vi "反控参数设置.vi"(8 "value time":timestamp, 9 "value float":sgl, 10 "设置参数":T2(ring)=enum."CODMn", 11 "设置类型":T1(ring)=enum."i13002") -> ()   [LabVIEW 2016]
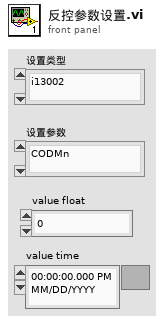
[diagram p1: front panel]
types:
  T1 = enum16{"i13001", "i13002", "i13003", "i13004", "i13005", "i13006", "i13007", "i13008", "i13009", "i13010", "i13011", "i13012", "i13013", "i13014", "i13015", "i13016", "i13017", "i13101", "i13102", "i13103", "i13104", "i13105", "i13106", "i13107", "i13108", "i13109", "i13110"}
  T2 = enum16{"", "CODMn", "PH", "氨氮", "总氮", "总磷", "CODCr", "电导率", "水温", "溶解氧", "浊度", "叶绿素", "藻密度", "ORP"}
  T3 = cluster{"status":bool, "代码":u16, "source":string}
  T4 = cluster{"测量量程":dbl, "测量精度":dbl, "测量间隔":dbl, "消解温度":dbl, "消解时长":dbl, "空白校准时间":timestamp, "曲线截距":dbl, "曲线斜率":dbl, "测量检出限":dbl, "测量信号值":dbl, "线性相关系数":dbl, "二次多项式系数":dbl, "标样校准时间":timestamp, "稀释倍数":dbl, "三项式系数":dbl, "空白标定系数":dbl, "量程系数":dbl, "F0/ORPA":dbl, "F1/ORPB":dbl, "F2/ORPK":dbl, "F3":dbl, "F4":dbl, "F5":dbl, "F6":dbl, "F7":dbl, "X0/滴定数":dbl, "量程":dbl}
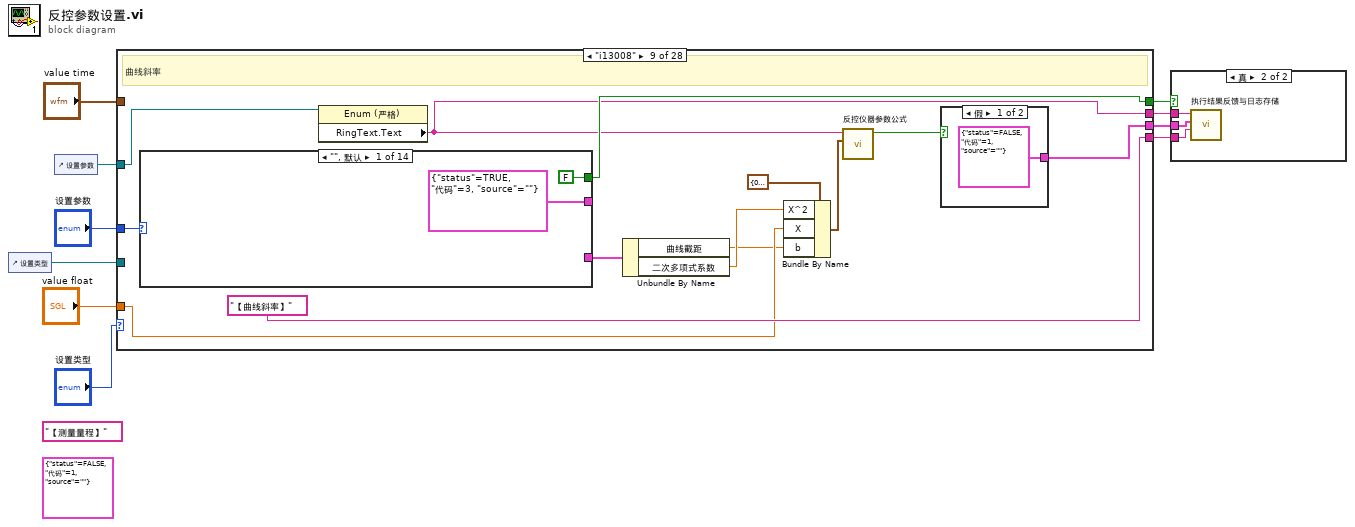
[diagram p0: block diagram]
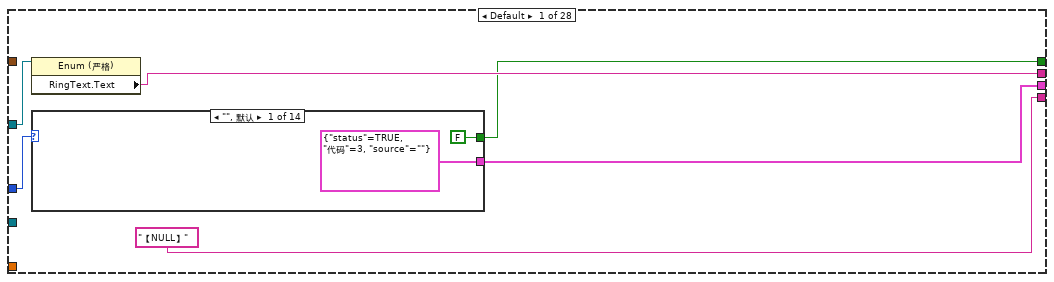
[diagram p3: hidden frame]
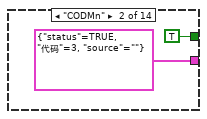
[diagram p4: hidden frame]
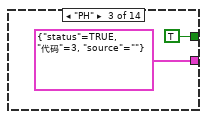
[diagram p5: hidden frame]
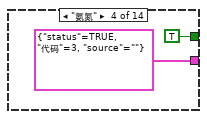
[diagram p6: hidden frame]
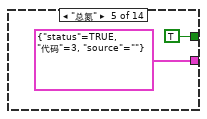
[diagram p7: hidden frame]
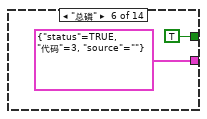
[diagram p8: hidden frame]
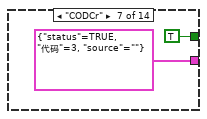
[diagram p9: hidden frame]
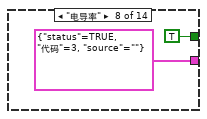
[diagram p10: hidden frame]
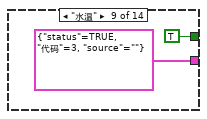
[diagram p11: hidden frame]
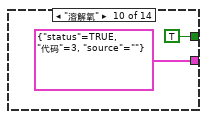
[diagram p12: hidden frame]
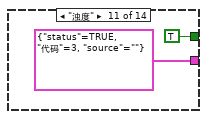
[diagram p13: hidden frame]
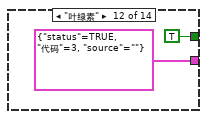
[diagram p14: hidden frame]
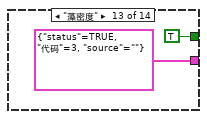
[diagram p15: hidden frame]
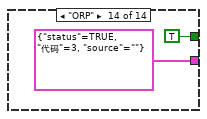
[diagram p16: hidden frame]
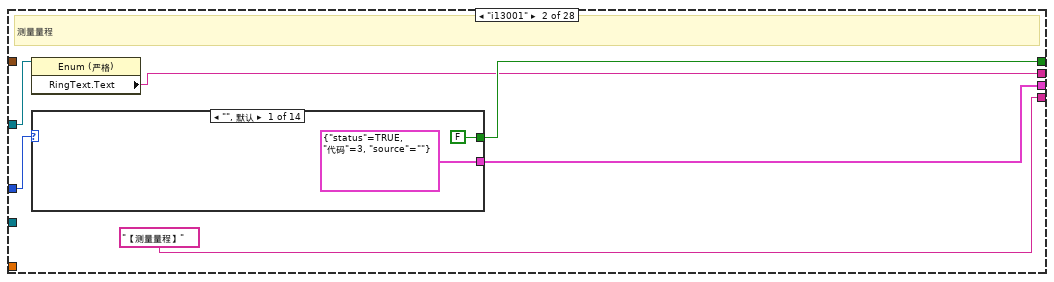
[diagram p17: hidden frame]
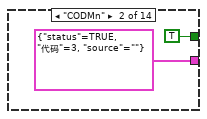
[diagram p18: hidden frame]
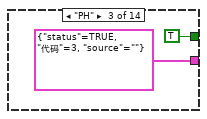
[diagram p19: hidden frame]
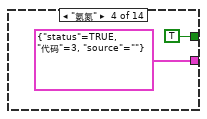
[diagram p20: hidden frame]
diagram:
  (unwired) T3 {"status"=FALSE, "代码"=1, "source"=""} ("error out")
  (unwired) "【测量量程】" ("日志信息")
  n1 = control-ref of="设置类型"() -> (w1:refnum<vi>)
  n2 = control-ref of="设置参数"() -> (w7:refnum<vi>)
  n3 = case shown="\"i13008\"" "设置类型" {
    tunnel: "设置参数" -> [w16 w50 w83 w114 w150 w193 w233 w277 w324 w363 w398 w434 w474 w513 w547 w581 w615 w649 w683 w717 w751 w789 w819 w853 w887 w921 w955 w989]
    tunnel: [w12 w49 w80 w116 w152 w196 w236 w279 w327 w366 w400 w432 w477 w516 w550 w584 w618 w652 w686 w720 w754 w786 w822 w856 w890 w924 w958 w992] -> w8
    tunnel: w7 -> [w15 w46 w84 w113 w154 w194 w234 w276 w325 w364 w397 w435 w475 w514 w548 w582 w616 w650 w684 w718 w752 w790 w820 w854 w888 w922 w956 w990]
    tunnel: [w14 w45 w82 w118 w149 w190 w238 w272 w318 w368 w402 w436 w468 w518 w552 w586 w620 w654 w688 w722 w756 w788 w824 w858 w892 w926 w960 w994] -> w6
    tunnel: ["【NULL】" ("日志信息") "【测量量程】" ("日志信息") "【测量精度】" ("日志信息") "【测量间隔】" ("日志信息") "【消解温度】" ("日志信息") "【消解时间】" ("日志信息") "【空白校准时间】" ("日志信息") "【曲线截距】" ("日志信息") "【曲线斜率】" ("日志信息") "【测量检出限】" ("日志信息") "【测量信号值】" ("日志信息") "【线性相关系数】" ("日志信息") "【二次项系数】" ("日志信息") "【标样校准时间】" ("日志信息") "【稀释倍数】" ("日志信息") "【三项式系数】" ("日志信息") "【空白标定系数】" ("日志信息") "【量程系数】" ("日志信息") "【F0/ORPA】" ("日志信息") "【F1/ORPB】" ("日志信息") "【F2/ORPK】" ("日志信息") "【F3】" ("日志信息") "【F4】" ("日志信息") "【F5】" ("日志信息") "【F6】" ("日志信息") "【F7】" ("日志信息") "【X0/滴定数】" ("日志信息") "【量程】" ("日志信息")] -> w5
    tunnel: [w13 w47 w81 w117 w153 w197 w237 w270 w320 w367 w401 w433 w470 w517 w551 w585 w619 w653 w687 w721 w755 w787 w823 w857 w891 w925 w959 w993] -> w4
    tunnel: "value float" -> [_ _ _ _ w148 w192 _ w273 w319 _ _ _ w469 _ _ _ _ _ _ _ _ _ _ _ _ _ _ _]
    tunnel: "value time" -> [_ _ _ _ _ _ _ _ _ _ _ _ _ _ _ _ _ _ _ _ _ _ _ _ _ _ _ _]
    tunnel: w1 -> [_ _ _ _ w147 w191 _ _ _ _ _ _ _ _ _ _ _ _ _ _ _ _ _ _ _ _ _ _]
    frame Default {
      n4 = property class="Enum (严格)"(reference=w15) -> ("RingText.Text"=w14:string)  [unwired: 1 in, 2 out]
      n5 = case shown="\"\", 默认" w16 {
        tunnel: [FALSE TRUE TRUE TRUE TRUE TRUE TRUE TRUE TRUE TRUE TRUE TRUE TRUE TRUE] -> w12
        tunnel: [T3 {"status"=TRUE, "代码"=3, "source"=""} ("error out") T3 {"status"=TRUE, "代码"=3, "source"=""} ("error out") T3 {"status"=TRUE, "代码"=3, "source"=""} ("error out") T3 {"status"=TRUE, "代码"=3, "source"=""} ("error out") T3 {"status"=TRUE, "代码"=3, "source"=""} ("error out") T3 {"status"=TRUE, "代码"=3, "source"=""} ("error out") T3 {"status"=TRUE, "代码"=3, "source"=""} ("error out") T3 {"status"=TRUE, "代码"=3, "source"=""} ("error out") T3 {"status"=TRUE, "代码"=3, "source"=""} ("error out") T3 {"status"=TRUE, "代码"=3, "source"=""} ("error out") T3 {"status"=TRUE, "代码"=3, "source"=""} ("error out") T3 {"status"=TRUE, "代码"=3, "source"=""} ("error out") T3 {"status"=TRUE, "代码"=3, "source"=""} ("error out") T3 {"status"=TRUE, "代码"=3, "source"=""} ("error out")] -> w13
        frame "", Default {
        }
        frame "CODMn" {
        }
        frame "PH" {
        }
        frame "氨氮" {
        }
        frame "总氮" {
        }
        frame "总磷" {
        }
        frame "CODCr" {
        }
        frame "电导率" {
        }
        frame "水温" {
        }
        frame "溶解氧" {
        }
        frame "浊度" {
        }
        frame "叶绿素" {
        }
        frame "藻密度" {
        }
        frame "ORP" {
        }
      }
    }
    frame "i13001" {
      # "测量量程"
      n6 = property class="Enum (严格)"(reference=w46) -> ("RingText.Text"=w45:string)  [unwired: 1 in, 2 out]
      n7 = case shown="\"\", 默认" w50 {
        tunnel: [FALSE TRUE TRUE TRUE TRUE TRUE TRUE TRUE TRUE TRUE TRUE TRUE TRUE TRUE] -> w49
        tunnel: [T3 {"status"=TRUE, "代码"=3, "source"=""} ("error out") T3 {"status"=TRUE, "代码"=3, "source"=""} ("error out") T3 {"status"=TRUE, "代码"=3, "source"=""} ("error out") T3 {"status"=TRUE, "代码"=3, "source"=""} ("error out") T3 {"status"=TRUE, "代码"=3, "source"=""} ("error out") T3 {"status"=TRUE, "代码"=3, "source"=""} ("error out") T3 {"status"=TRUE, "代码"=3, "source"=""} ("error out") T3 {"status"=TRUE, "代码"=3, "source"=""} ("error out") T3 {"status"=TRUE, "代码"=3, "source"=""} ("error out") T3 {"status"=TRUE, "代码"=3, "source"=""} ("error out") T3 {"status"=TRUE, "代码"=3, "source"=""} ("error out") T3 {"status"=TRUE, "代码"=3, "source"=""} ("error out") T3 {"status"=TRUE, "代码"=3, "source"=""} ("error out") T3 {"status"=TRUE, "代码"=3, "source"=""} ("error out")] -> w47
        frame "", Default {
        }
        frame "CODMn" {
        }
        frame "PH" {
        }
        frame "氨氮" {
        }
        frame "总氮" {
        }
        frame "总磷" {
        }
        frame "CODCr" {
        }
        frame "电导率" {
        }
        frame "水温" {
        }
        frame "溶解氧" {
        }
        frame "浊度" {
        }
        frame "叶绿素" {
        }
        frame "藻密度" {
        }
        frame "ORP" {
        }
      }
    }
    frame "i13002" {
      # "测量精度"
      n8 = property class="Enum (严格)"(reference=w84) -> ("RingText.Text"=w82:string)  [unwired: 1 in, 2 out]
      n9 = case shown="\"\", 默认" w83 {
        tunnel: [FALSE TRUE TRUE TRUE TRUE TRUE TRUE TRUE TRUE TRUE TRUE TRUE TRUE TRUE] -> w80
        tunnel: [T3 {"status"=TRUE, "代码"=3, "source"=""} ("error out") T3 {"status"=TRUE, "代码"=3, "source"=""} ("error out") T3 {"status"=TRUE, "代码"=3, "source"=""} ("error out") T3 {"status"=TRUE, "代码"=3, "source"=""} ("error out") T3 {"status"=TRUE, "代码"=3, "source"=""} ("error out") T3 {"status"=TRUE, "代码"=3, "source"=""} ("error out") T3 {"status"=TRUE, "代码"=3, "source"=""} ("error out") T3 {"status"=TRUE, "代码"=3, "source"=""} ("error out") T3 {"status"=TRUE, "代码"=3, "source"=""} ("error out") T3 {"status"=TRUE, "代码"=3, "source"=""} ("error out") T3 {"status"=TRUE, "代码"=3, "source"=""} ("error out") T3 {"status"=TRUE, "代码"=3, "source"=""} ("error out") T3 {"status"=TRUE, "代码"=3, "source"=""} ("error out") T3 {"status"=TRUE, "代码"=3, "source"=""} ("error out")] -> w81
        frame "", Default {
        }
        frame "CODMn" {
        }
        frame "PH" {
        }
        frame "氨氮" {
        }
        frame "总氮" {
        }
        frame "总磷" {
        }
        frame "CODCr" {
        }
        frame "电导率" {
        }
        frame "水温" {
        }
        frame "溶解氧" {
        }
        frame "浊度" {
        }
        frame "叶绿素" {
        }
        frame "藻密度" {
        }
        frame "ORP" {
        }
      }
    }
    frame "i13003" {
      # "测量间隔"
      n10 = property class="Enum (严格)"(reference=w113) -> ("RingText.Text"=w118:string)  [unwired: 1 in, 2 out]
      n11 = case shown="\"\", 默认" w114 {
        tunnel: [FALSE TRUE TRUE TRUE TRUE TRUE TRUE TRUE TRUE TRUE TRUE TRUE TRUE TRUE] -> w116
        tunnel: [T3 {"status"=TRUE, "代码"=3, "source"=""} ("error out") T3 {"status"=TRUE, "代码"=3, "source"=""} ("error out") T3 {"status"=TRUE, "代码"=3, "source"=""} ("error out") T3 {"status"=TRUE, "代码"=3, "source"=""} ("error out") T3 {"status"=TRUE, "代码"=3, "source"=""} ("error out") T3 {"status"=TRUE, "代码"=3, "source"=""} ("error out") T3 {"status"=TRUE, "代码"=3, "source"=""} ("error out") T3 {"status"=TRUE, "代码"=3, "source"=""} ("error out") T3 {"status"=TRUE, "代码"=3, "source"=""} ("error out") T3 {"status"=TRUE, "代码"=3, "source"=""} ("error out") T3 {"status"=TRUE, "代码"=3, "source"=""} ("error out") T3 {"status"=TRUE, "代码"=3, "source"=""} ("error out") T3 {"status"=TRUE, "代码"=3, "source"=""} ("error out") T3 {"status"=TRUE, "代码"=3, "source"=""} ("error out")] -> w117
        frame "", Default {
        }
        frame "CODMn" {
        }
        frame "PH" {
        }
        frame "氨氮" {
        }
        frame "总氮" {
        }
        frame "总磷" {
        }
        frame "CODCr" {
        }
        frame "电导率" {
        }
        frame "水温" {
        }
        frame "溶解氧" {
        }
        frame "浊度" {
        }
        frame "叶绿素" {
        }
        frame "藻密度" {
        }
        frame "ORP" {
        }
      }
    }
    frame "i13004" {
      # "消解温度"
      n12 = property class="Enum (严格)"(reference=w154) -> ("RingText.Text"=w149:string)  [unwired: 1 in, 2 out]
      n13 = case shown="\"CODMn\"" w150 {
        tunnel: [FALSE TRUE TRUE TRUE TRUE TRUE TRUE TRUE TRUE TRUE TRUE TRUE TRUE TRUE] -> w152
        tunnel: [T3 {"status"=TRUE, "代码"=3, "source"=""} ("error out") w159 T3 {"status"=TRUE, "代码"=3, "source"=""} ("error out") T3 {"status"=TRUE, "代码"=3, "source"=""} ("error out") T3 {"status"=TRUE, "代码"=3, "source"=""} ("error out") T3 {"status"=TRUE, "代码"=3, "source"=""} ("error out") T3 {"status"=TRUE, "代码"=3, "source"=""} ("error out") T3 {"status"=TRUE, "代码"=3, "source"=""} ("error out") T3 {"status"=TRUE, "代码"=3, "source"=""} ("error out") T3 {"status"=TRUE, "代码"=3, "source"=""} ("error out") T3 {"status"=TRUE, "代码"=3, "source"=""} ("error out") T3 {"status"=TRUE, "代码"=3, "source"=""} ("error out") T3 {"status"=TRUE, "代码"=3, "source"=""} ("error out") T3 {"status"=TRUE, "代码"=3, "source"=""} ("error out")] -> w153
        tunnel: w149 -> [_ w162 _ _ _ _ _ _ _ _ _ _ _ _]
        tunnel: w148 -> [_ w161 _ _ _ _ _ _ _ _ _ _ _ _]
        tunnel: w147 -> [_ w158 _ _ _ _ _ _ _ _ _ _ _ _]
        frame "", Default {
        }
        frame "CODMn" {
          n14 = property class="Enum (严格)"(reference=w158) -> ("RingText.Text"=w157:string)  [unwired: 1 in, 2 out]
          n15 = call "反控仪器单参数通用.vi"("参数"=w162, "value float"=w161, "chose"=w157) -> ("超时？"=w160:bool)  [unwired: 7 in, 1 out]
          n16 = case shown="假" w160 {
            tunnel: [T3 {"status"=FALSE, "代码"=1, "source"=""} ("error out") T3 {"status"=TRUE, "代码"=4, "source"=""} ("error out")] -> w159
            frame False {
            }
            frame True {
            }
          }
        }
        frame "PH" {
        }
        frame "氨氮" {
        }
        frame "总氮" {
        }
        frame "总磷" {
        }
        frame "CODCr" {
        }
        frame "电导率" {
        }
        frame "水温" {
        }
        frame "溶解氧" {
        }
        frame "浊度" {
        }
        frame "叶绿素" {
        }
        frame "藻密度" {
        }
        frame "ORP" {
        }
      }
    }
    frame "i13005" {
      # "消解时间"
      n17 = property class="Enum (严格)"(reference=w194) -> ("RingText.Text"=w190:string)  [unwired: 1 in, 2 out]
      n18 = case shown="\"CODMn\"" w193 {
        tunnel: [FALSE TRUE TRUE TRUE TRUE TRUE TRUE TRUE TRUE TRUE TRUE TRUE TRUE TRUE] -> w196
        tunnel: [T3 {"status"=TRUE, "代码"=3, "source"=""} ("error out") w200 T3 {"status"=TRUE, "代码"=3, "source"=""} ("error out") T3 {"status"=TRUE, "代码"=3, "source"=""} ("error out") T3 {"status"=TRUE, "代码"=3, "source"=""} ("error out") T3 {"status"=TRUE, "代码"=3, "source"=""} ("error out") T3 {"status"=TRUE, "代码"=3, "source"=""} ("error out") T3 {"status"=TRUE, "代码"=3, "source"=""} ("error out") T3 {"status"=TRUE, "代码"=3, "source"=""} ("error out") T3 {"status"=TRUE, "代码"=3, "source"=""} ("error out") T3 {"status"=TRUE, "代码"=3, "source"=""} ("error out") T3 {"status"=TRUE, "代码"=3, "source"=""} ("error out") T3 {"status"=TRUE, "代码"=3, "source"=""} ("error out") T3 {"status"=TRUE, "代码"=3, "source"=""} ("error out")] -> w197
        tunnel: w192 -> [_ w203 _ _ _ _ _ _ _ _ _ _ _ _]
        tunnel: w191 -> [_ w202 _ _ _ _ _ _ _ _ _ _ _ _]
        tunnel: w190 -> [_ w201 _ _ _ _ _ _ _ _ _ _ _ _]
        frame "", Default {
        }
        frame "CODMn" {
          n19 = property class="Enum (严格)"(reference=w202) -> ("RingText.Text"=w204:string)  [unwired: 1 in, 2 out]
          n20 = call "反控仪器单参数通用.vi"("参数"=w201, "value float"=w203, "chose"=w204) -> ("超时？"=w205:bool)  [unwired: 7 in, 1 out]
          n21 = case shown="假" w205 {
            tunnel: [T3 {"status"=FALSE, "代码"=1, "source"=""} ("error out") T3 {"status"=TRUE, "代码"=4, "source"=""} ("error out")] -> w200
            frame False {
            }
            frame True {
            }
          }
        }
        frame "PH" {
        }
        frame "氨氮" {
        }
        frame "总氮" {
        }
        frame "总磷" {
        }
        frame "CODCr" {
        }
        frame "电导率" {
        }
        frame "水温" {
        }
        frame "溶解氧" {
        }
        frame "浊度" {
        }
        frame "叶绿素" {
        }
        frame "藻密度" {
        }
        frame "ORP" {
        }
      }
    }
    frame "i13006" {
      # "空白校准时间"
      n22 = property class="Enum (严格)"(reference=w234) -> ("RingText.Text"=w238:string)  [unwired: 1 in, 2 out]
      n23 = case shown="\"\", 默认" w233 {
        tunnel: [FALSE TRUE TRUE TRUE TRUE TRUE TRUE TRUE TRUE TRUE TRUE TRUE TRUE TRUE] -> w236
        tunnel: [T3 {"status"=TRUE, "代码"=3, "source"=""} ("error out") T3 {"status"=TRUE, "代码"=3, "source"=""} ("error out") T3 {"status"=TRUE, "代码"=3, "source"=""} ("error out") T3 {"status"=TRUE, "代码"=3, "source"=""} ("error out") T3 {"status"=TRUE, "代码"=3, "source"=""} ("error out") T3 {"status"=TRUE, "代码"=3, "source"=""} ("error out") T3 {"status"=TRUE, "代码"=3, "source"=""} ("error out") T3 {"status"=TRUE, "代码"=3, "source"=""} ("error out") T3 {"status"=TRUE, "代码"=3, "source"=""} ("error out") T3 {"status"=TRUE, "代码"=3, "source"=""} ("error out") T3 {"status"=TRUE, "代码"=3, "source"=""} ("error out") T3 {"status"=TRUE, "代码"=3, "source"=""} ("error out") T3 {"status"=TRUE, "代码"=3, "source"=""} ("error out") T3 {"status"=TRUE, "代码"=3, "source"=""} ("error out")] -> w237
        frame "", Default {
        }
        frame "CODMn" {
        }
        frame "PH" {
        }
        frame "氨氮" {
        }
        frame "总氮" {
        }
        frame "总磷" {
        }
        frame "CODCr" {
        }
        frame "电导率" {
        }
        frame "水温" {
        }
        frame "溶解氧" {
        }
        frame "浊度" {
        }
        frame "叶绿素" {
        }
        frame "藻密度" {
        }
        frame "ORP" {
        }
      }
    }
    frame "i13007" {
      # "曲线截距"
      n24 = case shown="\"CODMn\"" w277 {
        tunnel: [FALSE TRUE TRUE TRUE TRUE TRUE TRUE TRUE TRUE TRUE TRUE TRUE TRUE TRUE] -> w279
        tunnel: [T3 {"status"=TRUE, "代码"=3, "source"=""} ("error out") T3 {"status"=TRUE, "代码"=3, "source"=""} ("error out") T3 {"status"=TRUE, "代码"=3, "source"=""} ("error out") T3 {"status"=TRUE, "代码"=3, "source"=""} ("error out") T3 {"status"=TRUE, "代码"=3, "source"=""} ("error out") T3 {"status"=TRUE, "代码"=3, "source"=""} ("error out") T3 {"status"=TRUE, "代码"=3, "source"=""} ("error out") T3 {"status"=TRUE, "代码"=3, "source"=""} ("error out") T3 {"status"=TRUE, "代码"=3, "source"=""} ("error out") T3 {"status"=TRUE, "代码"=3, "source"=""} ("error out") T3 {"status"=TRUE, "代码"=3, "source"=""} ("error out") T3 {"status"=TRUE, "代码"=3, "source"=""} ("error out") T3 {"status"=TRUE, "代码"=3, "source"=""} ("error out") T3 {"status"=TRUE, "代码"=3, "source"=""} ("error out")] -> _
        tunnel: [_ w284 _ w289 w292 w295 w298 _ _ _ _ _ _ _] -> w269
        frame "", Default {
        }
        frame "CODMn" {
          n25 = global read "CODMn断电保存全局变量.vi" "CODMn仪器参数"() -> (w284:T4)
        }
        frame "PH" {
        }
        frame "氨氮" {
          n26 = global read "总磷总氮断电保存全局变量.vi" "氨氮仪器参数"() -> (w289:T4)
        }
        frame "总氮" {
          n27 = global read "总磷总氮断电保存全局变量.vi" "总氮仪器参数"() -> (w292:T4)
        }
        frame "总磷" {
          n28 = global read "总磷总氮断电保存全局变量.vi" "总磷仪器参数"() -> (w295:T4)
        }
        frame "CODCr" {
          n29 = global read "CODcr全局变量.vi" "CODCr仪器参数"() -> (w298:T4)
        }
        frame "电导率" {
        }
        frame "水温" {
        }
        frame "溶解氧" {
        }
        frame "浊度" {
        }
        frame "叶绿素" {
        }
        frame "藻密度" {
        }
        frame "ORP" {
        }
      }
      n30 = property class="Enum (严格)"(reference=w276) -> ("RingText.Text"=w272:string)  [unwired: 1 in, 2 out]
      n31 = Unbundle By Name(w269) -> ("曲线斜率"=w268:dbl, "二次多项式系数"=w267:dbl)
      n32 = Bundle By Name(cluster=cluster{"X^2":dbl, "X":dbl, "b":dbl} {"X^2"=0.0, "X"=0.0, "b"=0.0} ("公式"), "X^2"=w267, "X"=w268, "b"=w273) -> (w275:cluster{"X^2":dbl, "X":dbl, "b":dbl})
      n33 = call "反控仪器参数公式.vi"("公式"=w275, "参数"=w272) -> ("超时？"=w271:bool)  [unwired: 8 in, 1 out]
      n34 = case shown="假" w271 {
        tunnel: [T3 {"status"=FALSE, "代码"=1, "source"=""} ("error out") T3 {"status"=TRUE, "代码"=4, "source"=""} ("error out")] -> w270
        frame False {
        }
        frame True {
        }
      }
    }
    frame "i13008" {
      # "曲线斜率"
      n35 = case shown="\"\", 默认" w324 {
        tunnel: [FALSE TRUE TRUE TRUE TRUE TRUE TRUE TRUE TRUE TRUE TRUE TRUE TRUE TRUE] -> w327
        tunnel: [T3 {"status"=TRUE, "代码"=3, "source"=""} ("error out") T3 {"status"=TRUE, "代码"=3, "source"=""} ("error out") T3 {"status"=TRUE, "代码"=3, "source"=""} ("error out") T3 {"status"=TRUE, "代码"=3, "source"=""} ("error out") T3 {"status"=TRUE, "代码"=3, "source"=""} ("error out") T3 {"status"=TRUE, "代码"=3, "source"=""} ("error out") T3 {"status"=TRUE, "代码"=3, "source"=""} ("error out") T3 {"status"=TRUE, "代码"=3, "source"=""} ("error out") T3 {"status"=TRUE, "代码"=3, "source"=""} ("error out") T3 {"status"=TRUE, "代码"=3, "source"=""} ("error out") T3 {"status"=TRUE, "代码"=3, "source"=""} ("error out") T3 {"status"=TRUE, "代码"=3, "source"=""} ("error out") T3 {"status"=TRUE, "代码"=3, "source"=""} ("error out") T3 {"status"=TRUE, "代码"=3, "source"=""} ("error out")] -> _
        tunnel: [_ w332 _ w337 w340 w343 w346 _ _ _ _ _ _ _] -> w315
        frame "", Default {
        }
        frame "CODMn" {
          n36 = global read "CODMn断电保存全局变量.vi" "CODMn仪器参数"() -> (w332:T4)
        }
        frame "PH" {
        }
        frame "氨氮" {
          n37 = global read "总磷总氮断电保存全局变量.vi" "氨氮仪器参数"() -> (w337:T4)
        }
        frame "总氮" {
          n38 = global read "总磷总氮断电保存全局变量.vi" "总氮仪器参数"() -> (w340:T4)
        }
        frame "总磷" {
          n39 = global read "总磷总氮断电保存全局变量.vi" "总磷仪器参数"() -> (w343:T4)
        }
        frame "CODCr" {
          n40 = global read "CODcr全局变量.vi" "CODCr仪器参数"() -> (w346:T4)
        }
        frame "电导率" {
        }
        frame "水温" {
        }
        frame "溶解氧" {
        }
        frame "浊度" {
        }
        frame "叶绿素" {
        }
        frame "藻密度" {
        }
        frame "ORP" {
        }
      }
      n41 = property class="Enum (严格)"(reference=w325) -> ("RingText.Text"=w318:string)  [unwired: 1 in, 2 out]
      n42 = Unbundle By Name(w315) -> ("曲线截距"=w316:dbl, "二次多项式系数"=w317:dbl)
      n43 = Bundle By Name(cluster=cluster{"X^2":dbl, "X":dbl, "b":dbl} {"X^2"=0.0, "X"=0.0, "b"=0.0} ("公式"), "X^2"=w317, "X"=w319, "b"=w316) -> (w321:cluster{"X^2":dbl, "X":dbl, "b":dbl})
      n44 = call "反控仪器参数公式.vi"("公式"=w321, "参数"=w318) -> ("超时？"=w323:bool)  [unwired: 8 in, 1 out]
      n45 = case shown="假" w323 {
        tunnel: [T3 {"status"=FALSE, "代码"=1, "source"=""} ("error out") T3 {"status"=TRUE, "代码"=4, "source"=""} ("error out")] -> w320
        frame False {
        }
        frame True {
        }
      }
    }
    frame "i13009" {
      # "测量检出限"
      n46 = property class="Enum (严格)"(reference=w364) -> ("RingText.Text"=w368:string)  [unwired: 1 in, 2 out]
      n47 = case shown="\"\", 默认" w363 {
        tunnel: [FALSE TRUE TRUE TRUE TRUE TRUE TRUE TRUE TRUE TRUE TRUE TRUE TRUE TRUE] -> w366
        tunnel: [T3 {"status"=TRUE, "代码"=3, "source"=""} ("error out") T3 {"status"=TRUE, "代码"=3, "source"=""} ("error out") T3 {"status"=TRUE, "代码"=3, "source"=""} ("error out") T3 {"status"=TRUE, "代码"=3, "source"=""} ("error out") T3 {"status"=TRUE, "代码"=3, "source"=""} ("error out") T3 {"status"=TRUE, "代码"=3, "source"=""} ("error out") T3 {"status"=TRUE, "代码"=3, "source"=""} ("error out") T3 {"status"=TRUE, "代码"=3, "source"=""} ("error out") T3 {"status"=TRUE, "代码"=3, "source"=""} ("error out") T3 {"status"=TRUE, "代码"=3, "source"=""} ("error out") T3 {"status"=TRUE, "代码"=3, "source"=""} ("error out") T3 {"status"=TRUE, "代码"=3, "source"=""} ("error out") T3 {"status"=TRUE, "代码"=3, "source"=""} ("error out") T3 {"status"=TRUE, "代码"=3, "source"=""} ("error out")] -> w367
        frame "", Default {
        }
        frame "CODMn" {
        }
        frame "PH" {
        }
        frame "氨氮" {
        }
        frame "总氮" {
        }
        frame "总磷" {
        }
        frame "CODCr" {
        }
        frame "电导率" {
        }
        frame "水温" {
        }
        frame "溶解氧" {
        }
        frame "浊度" {
        }
        frame "叶绿素" {
        }
        frame "藻密度" {
        }
        frame "ORP" {
        }
      }
    }
    frame "i13010" {
      # "测量信号值"
      n48 = property class="Enum (严格)"(reference=w397) -> ("RingText.Text"=w402:string)  [unwired: 1 in, 2 out]
      n49 = case shown="\"\", 默认" w398 {
        tunnel: [FALSE TRUE TRUE TRUE TRUE TRUE TRUE TRUE TRUE TRUE TRUE TRUE TRUE TRUE] -> w400
        tunnel: [T3 {"status"=TRUE, "代码"=3, "source"=""} ("error out") T3 {"status"=TRUE, "代码"=3, "source"=""} ("error out") T3 {"status"=TRUE, "代码"=3, "source"=""} ("error out") T3 {"status"=TRUE, "代码"=3, "source"=""} ("error out") T3 {"status"=TRUE, "代码"=3, "source"=""} ("error out") T3 {"status"=TRUE, "代码"=3, "source"=""} ("error out") T3 {"status"=TRUE, "代码"=3, "source"=""} ("error out") T3 {"status"=TRUE, "代码"=3, "source"=""} ("error out") T3 {"status"=TRUE, "代码"=3, "source"=""} ("error out") T3 {"status"=TRUE, "代码"=3, "source"=""} ("error out") T3 {"status"=TRUE, "代码"=3, "source"=""} ("error out") T3 {"status"=TRUE, "代码"=3, "source"=""} ("error out") T3 {"status"=TRUE, "代码"=3, "source"=""} ("error out") T3 {"status"=TRUE, "代码"=3, "source"=""} ("error out")] -> w401
        frame "", Default {
        }
        frame "CODMn" {
        }
        frame "PH" {
        }
        frame "氨氮" {
        }
        frame "总氮" {
        }
        frame "总磷" {
        }
        frame "CODCr" {
        }
        frame "电导率" {
        }
        frame "水温" {
        }
        frame "溶解氧" {
        }
        frame "浊度" {
        }
        frame "叶绿素" {
        }
        frame "藻密度" {
        }
        frame "ORP" {
        }
      }
    }
    frame "i13011" {
      # "线性相关系数"
      n50 = property class="Enum (严格)"(reference=w435) -> ("RingText.Text"=w436:string)  [unwired: 1 in, 2 out]
      n51 = case shown="\"\", 默认" w434 {
        tunnel: [FALSE TRUE TRUE TRUE TRUE TRUE TRUE TRUE TRUE TRUE TRUE TRUE TRUE TRUE] -> w432
        tunnel: [T3 {"status"=TRUE, "代码"=3, "source"=""} ("error out") T3 {"status"=TRUE, "代码"=3, "source"=""} ("error out") T3 {"status"=TRUE, "代码"=3, "source"=""} ("error out") T3 {"status"=TRUE, "代码"=3, "source"=""} ("error out") T3 {"status"=TRUE, "代码"=3, "source"=""} ("error out") T3 {"status"=TRUE, "代码"=3, "source"=""} ("error out") T3 {"status"=TRUE, "代码"=3, "source"=""} ("error out") T3 {"status"=TRUE, "代码"=3, "source"=""} ("error out") T3 {"status"=TRUE, "代码"=3, "source"=""} ("error out") T3 {"status"=TRUE, "代码"=3, "source"=""} ("error out") T3 {"status"=TRUE, "代码"=3, "source"=""} ("error out") T3 {"status"=TRUE, "代码"=3, "source"=""} ("error out") T3 {"status"=TRUE, "代码"=3, "source"=""} ("error out") T3 {"status"=TRUE, "代码"=3, "source"=""} ("error out")] -> w433
        frame "", Default {
        }
        frame "CODMn" {
        }
        frame "PH" {
        }
        frame "氨氮" {
        }
        frame "总氮" {
        }
        frame "总磷" {
        }
        frame "CODCr" {
        }
        frame "电导率" {
        }
        frame "水温" {
        }
        frame "溶解氧" {
        }
        frame "浊度" {
        }
        frame "叶绿素" {
        }
        frame "藻密度" {
        }
        frame "ORP" {
        }
      }
    }
    frame "i13012" {
      # "二次项系数"
      n52 = case shown="\"CODCr\"" w474 {
        tunnel: [FALSE TRUE TRUE TRUE TRUE TRUE TRUE TRUE TRUE TRUE TRUE TRUE TRUE TRUE] -> w477
        tunnel: [T3 {"status"=TRUE, "代码"=3, "source"=""} ("error out") T3 {"status"=TRUE, "代码"=3, "source"=""} ("error out") T3 {"status"=TRUE, "代码"=3, "source"=""} ("error out") T3 {"status"=TRUE, "代码"=3, "source"=""} ("error out") T3 {"status"=TRUE, "代码"=3, "source"=""} ("error out") T3 {"status"=TRUE, "代码"=3, "source"=""} ("error out") T3 {"status"=TRUE, "代码"=3, "source"=""} ("error out") T3 {"status"=TRUE, "代码"=3, "source"=""} ("error out") T3 {"status"=TRUE, "代码"=3, "source"=""} ("error out") T3 {"status"=TRUE, "代码"=3, "source"=""} ("error out") T3 {"status"=TRUE, "代码"=3, "source"=""} ("error out") T3 {"status"=TRUE, "代码"=3, "source"=""} ("error out") T3 {"status"=TRUE, "代码"=3, "source"=""} ("error out") T3 {"status"=TRUE, "代码"=3, "source"=""} ("error out")] -> _
        tunnel: [_ w482 _ w487 w490 w493 w496 _ _ _ _ _ _ _] -> w465
        frame "", Default {
        }
        frame "CODMn" {
          n53 = global read "CODMn断电保存全局变量.vi" "CODMn仪器参数"() -> (w482:T4)
        }
        frame "PH" {
        }
        frame "氨氮" {
          n54 = global read "总磷总氮断电保存全局变量.vi" "氨氮仪器参数"() -> (w487:T4)
        }
        frame "总氮" {
          n55 = global read "总磷总氮断电保存全局变量.vi" "总氮仪器参数"() -> (w490:T4)
        }
        frame "总磷" {
          n56 = global read "总磷总氮断电保存全局变量.vi" "总磷仪器参数"() -> (w493:T4)
        }
        frame "CODCr" {
          n57 = global read "CODcr全局变量.vi" "CODCr仪器参数"() -> (w496:T4)
        }
        frame "电导率" {
        }
        frame "水温" {
        }
        frame "溶解氧" {
        }
        frame "浊度" {
        }
        frame "叶绿素" {
        }
        frame "藻密度" {
        }
        frame "ORP" {
        }
      }
      n58 = property class="Enum (严格)"(reference=w475) -> ("RingText.Text"=w468:string)  [unwired: 1 in, 2 out]
      n59 = Unbundle By Name(w465) -> ("曲线截距"=w467:dbl, "曲线斜率"=w466:dbl)
      n60 = Bundle By Name(cluster=cluster{"X^2":dbl, "X":dbl, "b":dbl} {"X^2"=0.0, "X"=0.0, "b"=0.0} ("公式"), "X^2"=w469, "X"=w466, "b"=w467) -> (w471:cluster{"X^2":dbl, "X":dbl, "b":dbl})
      n61 = call "反控仪器参数公式.vi"("公式"=w471, "参数"=w468) -> ("超时？"=w473:bool)  [unwired: 8 in, 1 out]
      n62 = case shown="假" w473 {
        tunnel: [T3 {"status"=FALSE, "代码"=1, "source"=""} ("error out") T3 {"status"=TRUE, "代码"=4, "source"=""} ("error out")] -> w470
        frame False {
        }
        frame True {
        }
      }
    }
    frame "i13013" {
      # "标样校准时间"
      n63 = property class="Enum (严格)"(reference=w514) -> ("RingText.Text"=w518:string)  [unwired: 1 in, 2 out]
      n64 = case shown="\"CODMn\"" w513 {
        tunnel: [FALSE TRUE TRUE TRUE TRUE TRUE TRUE TRUE TRUE TRUE TRUE TRUE TRUE TRUE] -> w516
        tunnel: [T3 {"status"=TRUE, "代码"=3, "source"=""} ("error out") T3 {"status"=TRUE, "代码"=3, "source"=""} ("error out") T3 {"status"=TRUE, "代码"=3, "source"=""} ("error out") T3 {"status"=TRUE, "代码"=3, "source"=""} ("error out") T3 {"status"=TRUE, "代码"=3, "source"=""} ("error out") T3 {"status"=TRUE, "代码"=3, "source"=""} ("error out") T3 {"status"=TRUE, "代码"=3, "source"=""} ("error out") T3 {"status"=TRUE, "代码"=3, "source"=""} ("error out") T3 {"status"=TRUE, "代码"=3, "source"=""} ("error out") T3 {"status"=TRUE, "代码"=3, "source"=""} ("error out") T3 {"status"=TRUE, "代码"=3, "source"=""} ("error out") T3 {"status"=TRUE, "代码"=3, "source"=""} ("error out") T3 {"status"=TRUE, "代码"=3, "source"=""} ("error out") T3 {"status"=TRUE, "代码"=3, "source"=""} ("error out")] -> w517
        frame "", Default {
        }
        frame "CODMn" {
        }
        frame "PH" {
        }
        frame "氨氮" {
        }
        frame "总氮" {
        }
        frame "总磷" {
        }
        frame "CODCr" {
        }
        frame "电导率" {
        }
        frame "水温" {
        }
        frame "溶解氧" {
        }
        frame "浊度" {
        }
        frame "叶绿素" {
        }
        frame "藻密度" {
        }
        frame "ORP" {
        }
      }
    }
    frame "i13014" {
      # "稀释倍数"
      n65 = property class="Enum (严格)"(reference=w548) -> ("RingText.Text"=w552:string)  [unwired: 1 in, 2 out]
      n66 = case shown="\"\", 默认" w547 {
        tunnel: [FALSE TRUE TRUE TRUE TRUE TRUE TRUE TRUE TRUE TRUE TRUE TRUE TRUE TRUE] -> w550
        tunnel: [T3 {"status"=TRUE, "代码"=3, "source"=""} ("error out") T3 {"status"=TRUE, "代码"=3, "source"=""} ("error out") T3 {"status"=TRUE, "代码"=3, "source"=""} ("error out") T3 {"status"=TRUE, "代码"=3, "source"=""} ("error out") T3 {"status"=TRUE, "代码"=3, "source"=""} ("error out") T3 {"status"=TRUE, "代码"=3, "source"=""} ("error out") T3 {"status"=TRUE, "代码"=3, "source"=""} ("error out") T3 {"status"=TRUE, "代码"=3, "source"=""} ("error out") T3 {"status"=TRUE, "代码"=3, "source"=""} ("error out") T3 {"status"=TRUE, "代码"=3, "source"=""} ("error out") T3 {"status"=TRUE, "代码"=3, "source"=""} ("error out") T3 {"status"=TRUE, "代码"=3, "source"=""} ("error out") T3 {"status"=TRUE, "代码"=3, "source"=""} ("error out") T3 {"status"=TRUE, "代码"=3, "source"=""} ("error out")] -> w551
        frame "", Default {
        }
        frame "CODMn" {
        }
        frame "PH" {
        }
        frame "氨氮" {
        }
        frame "总氮" {
        }
        frame "总磷" {
        }
        frame "CODCr" {
        }
        frame "电导率" {
        }
        frame "水温" {
        }
        frame "溶解氧" {
        }
        frame "浊度" {
        }
        frame "叶绿素" {
        }
        frame "藻密度" {
        }
        frame "ORP" {
        }
      }
    }
    frame "i13015" {
      # "三项式系数"
      n67 = property class="Enum (严格)"(reference=w582) -> ("RingText.Text"=w586:string)  [unwired: 1 in, 2 out]
      n68 = case shown="\"\", 默认" w581 {
        tunnel: [FALSE TRUE TRUE TRUE TRUE TRUE TRUE TRUE TRUE TRUE TRUE TRUE TRUE TRUE] -> w584
        tunnel: [T3 {"status"=TRUE, "代码"=3, "source"=""} ("error out") T3 {"status"=TRUE, "代码"=3, "source"=""} ("error out") T3 {"status"=TRUE, "代码"=3, "source"=""} ("error out") T3 {"status"=TRUE, "代码"=3, "source"=""} ("error out") T3 {"status"=TRUE, "代码"=3, "source"=""} ("error out") T3 {"status"=TRUE, "代码"=3, "source"=""} ("error out") T3 {"status"=TRUE, "代码"=3, "source"=""} ("error out") T3 {"status"=TRUE, "代码"=3, "source"=""} ("error out") T3 {"status"=TRUE, "代码"=3, "source"=""} ("error out") T3 {"status"=TRUE, "代码"=3, "source"=""} ("error out") T3 {"status"=TRUE, "代码"=3, "source"=""} ("error out") T3 {"status"=TRUE, "代码"=3, "source"=""} ("error out") T3 {"status"=TRUE, "代码"=3, "source"=""} ("error out") T3 {"status"=TRUE, "代码"=3, "source"=""} ("error out")] -> w585
        frame "", Default {
        }
        frame "CODMn" {
        }
        frame "PH" {
        }
        frame "氨氮" {
        }
        frame "总氮" {
        }
        frame "总磷" {
        }
        frame "CODCr" {
        }
        frame "电导率" {
        }
        frame "水温" {
        }
        frame "溶解氧" {
        }
        frame "浊度" {
        }
        frame "叶绿素" {
        }
        frame "藻密度" {
        }
        frame "ORP" {
        }
      }
    }
    frame "i13016" {
      # "空白标定系数"
      n69 = property class="Enum (严格)"(reference=w616) -> ("RingText.Text"=w620:string)  [unwired: 1 in, 2 out]
      n70 = case shown="\"\", 默认" w615 {
        tunnel: [FALSE TRUE TRUE TRUE TRUE TRUE TRUE TRUE TRUE TRUE TRUE TRUE TRUE TRUE] -> w618
        tunnel: [T3 {"status"=TRUE, "代码"=3, "source"=""} ("error out") T3 {"status"=TRUE, "代码"=3, "source"=""} ("error out") T3 {"status"=TRUE, "代码"=3, "source"=""} ("error out") T3 {"status"=TRUE, "代码"=3, "source"=""} ("error out") T3 {"status"=TRUE, "代码"=3, "source"=""} ("error out") T3 {"status"=TRUE, "代码"=3, "source"=""} ("error out") T3 {"status"=TRUE, "代码"=3, "source"=""} ("error out") T3 {"status"=TRUE, "代码"=3, "source"=""} ("error out") T3 {"status"=TRUE, "代码"=3, "source"=""} ("error out") T3 {"status"=TRUE, "代码"=3, "source"=""} ("error out") T3 {"status"=TRUE, "代码"=3, "source"=""} ("error out") T3 {"status"=TRUE, "代码"=3, "source"=""} ("error out") T3 {"status"=TRUE, "代码"=3, "source"=""} ("error out") T3 {"status"=TRUE, "代码"=3, "source"=""} ("error out")] -> w619
        frame "", Default {
        }
        frame "CODMn" {
        }
        frame "PH" {
        }
        frame "氨氮" {
        }
        frame "总氮" {
        }
        frame "总磷" {
        }
        frame "CODCr" {
        }
        frame "电导率" {
        }
        frame "水温" {
        }
        frame "溶解氧" {
        }
        frame "浊度" {
        }
        frame "叶绿素" {
        }
        frame "藻密度" {
        }
        frame "ORP" {
        }
      }
    }
    frame "i13017" {
      # "量程系数"
      n71 = property class="Enum (严格)"(reference=w650) -> ("RingText.Text"=w654:string)  [unwired: 1 in, 2 out]
      n72 = case shown="\"\", 默认" w649 {
        tunnel: [FALSE TRUE TRUE TRUE TRUE TRUE TRUE TRUE TRUE TRUE TRUE TRUE TRUE TRUE] -> w652
        tunnel: [T3 {"status"=TRUE, "代码"=3, "source"=""} ("error out") T3 {"status"=TRUE, "代码"=3, "source"=""} ("error out") T3 {"status"=TRUE, "代码"=3, "source"=""} ("error out") T3 {"status"=TRUE, "代码"=3, "source"=""} ("error out") T3 {"status"=TRUE, "代码"=3, "source"=""} ("error out") T3 {"status"=TRUE, "代码"=3, "source"=""} ("error out") T3 {"status"=TRUE, "代码"=3, "source"=""} ("error out") T3 {"status"=TRUE, "代码"=3, "source"=""} ("error out") T3 {"status"=TRUE, "代码"=3, "source"=""} ("error out") T3 {"status"=TRUE, "代码"=3, "source"=""} ("error out") T3 {"status"=TRUE, "代码"=3, "source"=""} ("error out") T3 {"status"=TRUE, "代码"=3, "source"=""} ("error out") T3 {"status"=TRUE, "代码"=3, "source"=""} ("error out") T3 {"status"=TRUE, "代码"=3, "source"=""} ("error out")] -> w653
        frame "", Default {
        }
        frame "CODMn" {
        }
        frame "PH" {
        }
        frame "氨氮" {
        }
        frame "总氮" {
        }
        frame "总磷" {
        }
        frame "CODCr" {
        }
        frame "电导率" {
        }
        frame "水温" {
        }
        frame "溶解氧" {
        }
        frame "浊度" {
        }
        frame "叶绿素" {
        }
        frame "藻密度" {
        }
        frame "ORP" {
        }
      }
    }
    frame "i13101" {
      # "F0/ORPA"
      n73 = property class="Enum (严格)"(reference=w684) -> ("RingText.Text"=w688:string)  [unwired: 1 in, 2 out]
      n74 = case shown="\"\", 默认" w683 {
        tunnel: [FALSE TRUE TRUE TRUE TRUE TRUE TRUE TRUE TRUE TRUE TRUE TRUE TRUE TRUE] -> w686
        tunnel: [T3 {"status"=TRUE, "代码"=3, "source"=""} ("error out") T3 {"status"=TRUE, "代码"=3, "source"=""} ("error out") T3 {"status"=TRUE, "代码"=3, "source"=""} ("error out") T3 {"status"=TRUE, "代码"=3, "source"=""} ("error out") T3 {"status"=TRUE, "代码"=3, "source"=""} ("error out") T3 {"status"=TRUE, "代码"=3, "source"=""} ("error out") T3 {"status"=TRUE, "代码"=3, "source"=""} ("error out") T3 {"status"=TRUE, "代码"=3, "source"=""} ("error out") T3 {"status"=TRUE, "代码"=3, "source"=""} ("error out") T3 {"status"=TRUE, "代码"=3, "source"=""} ("error out") T3 {"status"=TRUE, "代码"=3, "source"=""} ("error out") T3 {"status"=TRUE, "代码"=3, "source"=""} ("error out") T3 {"status"=TRUE, "代码"=3, "source"=""} ("error out") T3 {"status"=TRUE, "代码"=3, "source"=""} ("error out")] -> w687
        frame "", Default {
        }
        frame "CODMn" {
        }
        frame "PH" {
        }
        frame "氨氮" {
        }
        frame "总氮" {
        }
        frame "总磷" {
        }
        frame "CODCr" {
        }
        frame "电导率" {
        }
        frame "水温" {
        }
        frame "溶解氧" {
        }
        frame "浊度" {
        }
        frame "叶绿素" {
        }
        frame "藻密度" {
        }
        frame "ORP" {
        }
      }
    }
    frame "i13102" {
      # "F1/ORPB"
      n75 = property class="Enum (严格)"(reference=w718) -> ("RingText.Text"=w722:string)  [unwired: 1 in, 2 out]
      n76 = case shown="\"\", 默认" w717 {
        tunnel: [FALSE TRUE TRUE TRUE TRUE TRUE TRUE TRUE TRUE TRUE TRUE TRUE TRUE TRUE] -> w720
        tunnel: [T3 {"status"=TRUE, "代码"=3, "source"=""} ("error out") T3 {"status"=TRUE, "代码"=3, "source"=""} ("error out") T3 {"status"=TRUE, "代码"=3, "source"=""} ("error out") T3 {"status"=TRUE, "代码"=3, "source"=""} ("error out") T3 {"status"=TRUE, "代码"=3, "source"=""} ("error out") T3 {"status"=TRUE, "代码"=3, "source"=""} ("error out") T3 {"status"=TRUE, "代码"=3, "source"=""} ("error out") T3 {"status"=TRUE, "代码"=3, "source"=""} ("error out") T3 {"status"=TRUE, "代码"=3, "source"=""} ("error out") T3 {"status"=TRUE, "代码"=3, "source"=""} ("error out") T3 {"status"=TRUE, "代码"=3, "source"=""} ("error out") T3 {"status"=TRUE, "代码"=3, "source"=""} ("error out") T3 {"status"=TRUE, "代码"=3, "source"=""} ("error out") T3 {"status"=TRUE, "代码"=3, "source"=""} ("error out")] -> w721
        frame "", Default {
        }
        frame "CODMn" {
        }
        frame "PH" {
        }
        frame "氨氮" {
        }
        frame "总氮" {
        }
        frame "总磷" {
        }
        frame "CODCr" {
        }
        frame "电导率" {
        }
        frame "水温" {
        }
        frame "溶解氧" {
        }
        frame "浊度" {
        }
        frame "叶绿素" {
        }
        frame "藻密度" {
        }
        frame "ORP" {
        }
      }
    }
    frame "i13103" {
      # "F2/ORPK"
      n77 = property class="Enum (严格)"(reference=w752) -> ("RingText.Text"=w756:string)  [unwired: 1 in, 2 out]
      n78 = case shown="\"\", 默认" w751 {
        tunnel: [FALSE TRUE TRUE TRUE TRUE TRUE TRUE TRUE TRUE TRUE TRUE TRUE TRUE TRUE] -> w754
        tunnel: [T3 {"status"=TRUE, "代码"=3, "source"=""} ("error out") T3 {"status"=TRUE, "代码"=3, "source"=""} ("error out") T3 {"status"=TRUE, "代码"=3, "source"=""} ("error out") T3 {"status"=TRUE, "代码"=3, "source"=""} ("error out") T3 {"status"=TRUE, "代码"=3, "source"=""} ("error out") T3 {"status"=TRUE, "代码"=3, "source"=""} ("error out") T3 {"status"=TRUE, "代码"=3, "source"=""} ("error out") T3 {"status"=TRUE, "代码"=3, "source"=""} ("error out") T3 {"status"=TRUE, "代码"=3, "source"=""} ("error out") T3 {"status"=TRUE, "代码"=3, "source"=""} ("error out") T3 {"status"=TRUE, "代码"=3, "source"=""} ("error out") T3 {"status"=TRUE, "代码"=3, "source"=""} ("error out") T3 {"status"=TRUE, "代码"=3, "source"=""} ("error out") T3 {"status"=TRUE, "代码"=3, "source"=""} ("error out")] -> w755
        frame "", Default {
        }
        frame "CODMn" {
        }
        frame "PH" {
        }
        frame "氨氮" {
        }
        frame "总氮" {
        }
        frame "总磷" {
        }
        frame "CODCr" {
        }
        frame "电导率" {
        }
        frame "水温" {
        }
        frame "溶解氧" {
        }
        frame "浊度" {
        }
        frame "叶绿素" {
        }
        frame "藻密度" {
        }
        frame "ORP" {
        }
      }
    }
    frame "i13104" {
      # "F3"
      n79 = property class="Enum (严格)"(reference=w790) -> ("RingText.Text"=w788:string)  [unwired: 1 in, 2 out]
      n80 = case shown="\"\", 默认" w789 {
        tunnel: [FALSE TRUE TRUE TRUE TRUE TRUE TRUE TRUE TRUE TRUE TRUE TRUE TRUE TRUE] -> w786
        tunnel: [T3 {"status"=TRUE, "代码"=3, "source"=""} ("error out") T3 {"status"=TRUE, "代码"=3, "source"=""} ("error out") T3 {"status"=TRUE, "代码"=3, "source"=""} ("error out") T3 {"status"=TRUE, "代码"=3, "source"=""} ("error out") T3 {"status"=TRUE, "代码"=3, "source"=""} ("error out") T3 {"status"=TRUE, "代码"=3, "source"=""} ("error out") T3 {"status"=TRUE, "代码"=3, "source"=""} ("error out") T3 {"status"=TRUE, "代码"=3, "source"=""} ("error out") T3 {"status"=TRUE, "代码"=3, "source"=""} ("error out") T3 {"status"=TRUE, "代码"=3, "source"=""} ("error out") T3 {"status"=TRUE, "代码"=3, "source"=""} ("error out") T3 {"status"=TRUE, "代码"=3, "source"=""} ("error out") T3 {"status"=TRUE, "代码"=3, "source"=""} ("error out") T3 {"status"=TRUE, "代码"=3, "source"=""} ("error out")] -> w787
        frame "", Default {
        }
        frame "CODMn" {
        }
        frame "PH" {
        }
        frame "氨氮" {
        }
        frame "总氮" {
        }
        frame "总磷" {
        }
        frame "CODCr" {
        }
        frame "电导率" {
        }
        frame "水温" {
        }
        frame "溶解氧" {
        }
        frame "浊度" {
        }
        frame "叶绿素" {
        }
        frame "藻密度" {
        }
        frame "ORP" {
        }
      }
    }
    frame "i13105" {
      # "F4"
      n81 = property class="Enum (严格)"(reference=w820) -> ("RingText.Text"=w824:string)  [unwired: 1 in, 2 out]
      n82 = case shown="\"\", 默认" w819 {
        tunnel: [FALSE TRUE TRUE TRUE TRUE TRUE TRUE TRUE TRUE TRUE TRUE TRUE TRUE TRUE] -> w822
        tunnel: [T3 {"status"=TRUE, "代码"=3, "source"=""} ("error out") T3 {"status"=TRUE, "代码"=3, "source"=""} ("error out") T3 {"status"=TRUE, "代码"=3, "source"=""} ("error out") T3 {"status"=TRUE, "代码"=3, "source"=""} ("error out") T3 {"status"=TRUE, "代码"=3, "source"=""} ("error out") T3 {"status"=TRUE, "代码"=3, "source"=""} ("error out") T3 {"status"=TRUE, "代码"=3, "source"=""} ("error out") T3 {"status"=TRUE, "代码"=3, "source"=""} ("error out") T3 {"status"=TRUE, "代码"=3, "source"=""} ("error out") T3 {"status"=TRUE, "代码"=3, "source"=""} ("error out") T3 {"status"=TRUE, "代码"=3, "source"=""} ("error out") T3 {"status"=TRUE, "代码"=3, "source"=""} ("error out") T3 {"status"=TRUE, "代码"=3, "source"=""} ("error out") T3 {"status"=TRUE, "代码"=3, "source"=""} ("error out")] -> w823
        frame "", Default {
        }
        frame "CODMn" {
        }
        frame "PH" {
        }
        frame "氨氮" {
        }
        frame "总氮" {
        }
        frame "总磷" {
        }
        frame "CODCr" {
        }
        frame "电导率" {
        }
        frame "水温" {
        }
        frame "溶解氧" {
        }
        frame "浊度" {
        }
        frame "叶绿素" {
        }
        frame "藻密度" {
        }
        frame "ORP" {
        }
      }
    }
    frame "i13106" {
      # "F5"
      n83 = property class="Enum (严格)"(reference=w854) -> ("RingText.Text"=w858:string)  [unwired: 1 in, 2 out]
      n84 = case shown="\"\", 默认" w853 {
        tunnel: [FALSE TRUE TRUE TRUE TRUE TRUE TRUE TRUE TRUE TRUE TRUE TRUE TRUE TRUE] -> w856
        tunnel: [T3 {"status"=TRUE, "代码"=3, "source"=""} ("error out") T3 {"status"=TRUE, "代码"=3, "source"=""} ("error out") T3 {"status"=TRUE, "代码"=3, "source"=""} ("error out") T3 {"status"=TRUE, "代码"=3, "source"=""} ("error out") T3 {"status"=TRUE, "代码"=3, "source"=""} ("error out") T3 {"status"=TRUE, "代码"=3, "source"=""} ("error out") T3 {"status"=TRUE, "代码"=3, "source"=""} ("error out") T3 {"status"=TRUE, "代码"=3, "source"=""} ("error out") T3 {"status"=TRUE, "代码"=3, "source"=""} ("error out") T3 {"status"=TRUE, "代码"=3, "source"=""} ("error out") T3 {"status"=TRUE, "代码"=3, "source"=""} ("error out") T3 {"status"=TRUE, "代码"=3, "source"=""} ("error out") T3 {"status"=TRUE, "代码"=3, "source"=""} ("error out") T3 {"status"=TRUE, "代码"=3, "source"=""} ("error out")] -> w857
        frame "", Default {
        }
        frame "CODMn" {
        }
        frame "PH" {
        }
        frame "氨氮" {
        }
        frame "总氮" {
        }
        frame "总磷" {
        }
        frame "CODCr" {
        }
        frame "电导率" {
        }
        frame "水温" {
        }
        frame "溶解氧" {
        }
        frame "浊度" {
        }
        frame "叶绿素" {
        }
        frame "藻密度" {
        }
        frame "ORP" {
        }
      }
    }
    frame "i13107" {
      # "F6"
      n85 = property class="Enum (严格)"(reference=w888) -> ("RingText.Text"=w892:string)  [unwired: 1 in, 2 out]
      n86 = case shown="\"\", 默认" w887 {
        tunnel: [FALSE TRUE TRUE TRUE TRUE TRUE TRUE TRUE TRUE TRUE TRUE TRUE TRUE TRUE] -> w890
        tunnel: [T3 {"status"=TRUE, "代码"=3, "source"=""} ("error out") T3 {"status"=TRUE, "代码"=3, "source"=""} ("error out") T3 {"status"=TRUE, "代码"=3, "source"=""} ("error out") T3 {"status"=TRUE, "代码"=3, "source"=""} ("error out") T3 {"status"=TRUE, "代码"=3, "source"=""} ("error out") T3 {"status"=TRUE, "代码"=3, "source"=""} ("error out") T3 {"status"=TRUE, "代码"=3, "source"=""} ("error out") T3 {"status"=TRUE, "代码"=3, "source"=""} ("error out") T3 {"status"=TRUE, "代码"=3, "source"=""} ("error out") T3 {"status"=TRUE, "代码"=3, "source"=""} ("error out") T3 {"status"=TRUE, "代码"=3, "source"=""} ("error out") T3 {"status"=TRUE, "代码"=3, "source"=""} ("error out") T3 {"status"=TRUE, "代码"=3, "source"=""} ("error out") T3 {"status"=TRUE, "代码"=3, "source"=""} ("error out")] -> w891
        frame "", Default {
        }
        frame "CODMn" {
        }
        frame "PH" {
        }
        frame "氨氮" {
        }
        frame "总氮" {
        }
        frame "总磷" {
        }
        frame "CODCr" {
        }
        frame "电导率" {
        }
        frame "水温" {
        }
        frame "溶解氧" {
        }
        frame "浊度" {
        }
        frame "叶绿素" {
        }
        frame "藻密度" {
        }
        frame "ORP" {
        }
      }
    }
    frame "i13108" {
      # "F7"
      n87 = property class="Enum (严格)"(reference=w922) -> ("RingText.Text"=w926:string)  [unwired: 1 in, 2 out]
      n88 = case shown="\"\", 默认" w921 {
        tunnel: [FALSE TRUE TRUE TRUE TRUE TRUE TRUE TRUE TRUE TRUE TRUE TRUE TRUE TRUE] -> w924
        tunnel: [T3 {"status"=TRUE, "代码"=3, "source"=""} ("error out") T3 {"status"=TRUE, "代码"=3, "source"=""} ("error out") T3 {"status"=TRUE, "代码"=3, "source"=""} ("error out") T3 {"status"=TRUE, "代码"=3, "source"=""} ("error out") T3 {"status"=TRUE, "代码"=3, "source"=""} ("error out") T3 {"status"=TRUE, "代码"=3, "source"=""} ("error out") T3 {"status"=TRUE, "代码"=3, "source"=""} ("error out") T3 {"status"=TRUE, "代码"=3, "source"=""} ("error out") T3 {"status"=TRUE, "代码"=3, "source"=""} ("error out") T3 {"status"=TRUE, "代码"=3, "source"=""} ("error out") T3 {"status"=TRUE, "代码"=3, "source"=""} ("error out") T3 {"status"=TRUE, "代码"=3, "source"=""} ("error out") T3 {"status"=TRUE, "代码"=3, "source"=""} ("error out") T3 {"status"=TRUE, "代码"=3, "source"=""} ("error out")] -> w925
        frame "", Default {
        }
        frame "CODMn" {
        }
        frame "PH" {
        }
        frame "氨氮" {
        }
        frame "总氮" {
        }
        frame "总磷" {
        }
        frame "CODCr" {
        }
        frame "电导率" {
        }
        frame "水温" {
        }
        frame "溶解氧" {
        }
        frame "浊度" {
        }
        frame "叶绿素" {
        }
        frame "藻密度" {
        }
        frame "ORP" {
        }
      }
    }
    frame "i13109" {
      # "X0/滴定数"
      n89 = property class="Enum (严格)"(reference=w956) -> ("RingText.Text"=w960:string)  [unwired: 1 in, 2 out]
      n90 = case shown="\"\", 默认" w955 {
        tunnel: [FALSE TRUE TRUE TRUE TRUE TRUE TRUE TRUE TRUE TRUE TRUE TRUE TRUE TRUE] -> w958
        tunnel: [T3 {"status"=TRUE, "代码"=3, "source"=""} ("error out") T3 {"status"=TRUE, "代码"=3, "source"=""} ("error out") T3 {"status"=TRUE, "代码"=3, "source"=""} ("error out") T3 {"status"=TRUE, "代码"=3, "source"=""} ("error out") T3 {"status"=TRUE, "代码"=3, "source"=""} ("error out") T3 {"status"=TRUE, "代码"=3, "source"=""} ("error out") T3 {"status"=TRUE, "代码"=3, "source"=""} ("error out") T3 {"status"=TRUE, "代码"=3, "source"=""} ("error out") T3 {"status"=TRUE, "代码"=3, "source"=""} ("error out") T3 {"status"=TRUE, "代码"=3, "source"=""} ("error out") T3 {"status"=TRUE, "代码"=3, "source"=""} ("error out") T3 {"status"=TRUE, "代码"=3, "source"=""} ("error out") T3 {"status"=TRUE, "代码"=3, "source"=""} ("error out") T3 {"status"=TRUE, "代码"=3, "source"=""} ("error out")] -> w959
        frame "", Default {
        }
        frame "CODMn" {
        }
        frame "PH" {
        }
        frame "氨氮" {
        }
        frame "总氮" {
        }
        frame "总磷" {
        }
        frame "CODCr" {
        }
        frame "电导率" {
        }
        frame "水温" {
        }
        frame "溶解氧" {
        }
        frame "浊度" {
        }
        frame "叶绿素" {
        }
        frame "藻密度" {
        }
        frame "ORP" {
        }
      }
    }
    frame "i13110" {
      # "量程"
      n91 = property class="Enum (严格)"(reference=w990) -> ("RingText.Text"=w994:string)  [unwired: 1 in, 2 out]
      n92 = case shown="\"\", 默认" w989 {
        tunnel: [FALSE TRUE TRUE TRUE TRUE TRUE TRUE TRUE TRUE TRUE TRUE TRUE TRUE TRUE] -> w992
        tunnel: [T3 {"status"=TRUE, "代码"=3, "source"=""} ("error out") T3 {"status"=TRUE, "代码"=3, "source"=""} ("error out") T3 {"status"=TRUE, "代码"=3, "source"=""} ("error out") T3 {"status"=TRUE, "代码"=3, "source"=""} ("error out") T3 {"status"=TRUE, "代码"=3, "source"=""} ("error out") T3 {"status"=TRUE, "代码"=3, "source"=""} ("error out") T3 {"status"=TRUE, "代码"=3, "source"=""} ("error out") T3 {"status"=TRUE, "代码"=3, "source"=""} ("error out") T3 {"status"=TRUE, "代码"=3, "source"=""} ("error out") T3 {"status"=TRUE, "代码"=3, "source"=""} ("error out") T3 {"status"=TRUE, "代码"=3, "source"=""} ("error out") T3 {"status"=TRUE, "代码"=3, "source"=""} ("error out") T3 {"status"=TRUE, "代码"=3, "source"=""} ("error out") T3 {"status"=TRUE, "代码"=3, "source"=""} ("error out")] -> w993
        frame "", Default {
        }
        frame "CODMn" {
        }
        frame "PH" {
        }
        frame "氨氮" {
        }
        frame "总氮" {
        }
        frame "总磷" {
        }
        frame "CODCr" {
        }
        frame "电导率" {
        }
        frame "水温" {
        }
        frame "溶解氧" {
        }
        frame "浊度" {
        }
        frame "叶绿素" {
        }
        frame "藻密度" {
        }
        frame "ORP" {
        }
      }
    }
  }
  n93 = case shown="真" w8 {
    tunnel: w6 -> [_ w1025]
    tunnel: w5 -> [_ w1024]
    tunnel: w4 -> [_ w1023]
    frame False {
    }
    frame True {
      n94 = call "执行结果反馈与日志存储.vi"("日志信息"=w1024, "error out"=w1023, "设备"=w1025) -> ()  [unwired: 9 in]
    }
  }
